vi "ASK_Channelcode.vi"(4 "k":i32, 6 "n":i32, 7 "cod_mode":i32, 8 "error in (no error)":errorcluster caption="错误输入（无错误）", 9 "生产多项式":dbl[](array[numeric]) format="%#_13g", 10 "CRC_Bit":dbl[](array[numeric]) format="%#_13g", 11 "PathIn":path) -> (0 "error out":errorcluster caption="错误输出", 2 "Channel_Bit":dbl[](array[numeric]), 3 "PathOut":path)   [LabVIEW 2015]
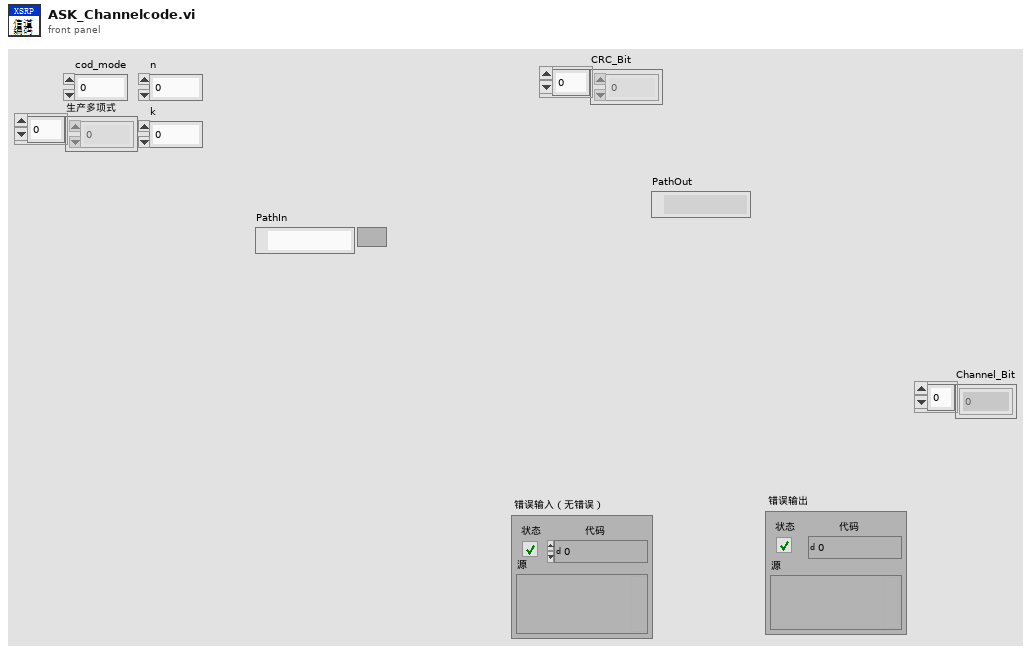
[diagram p1: front panel]
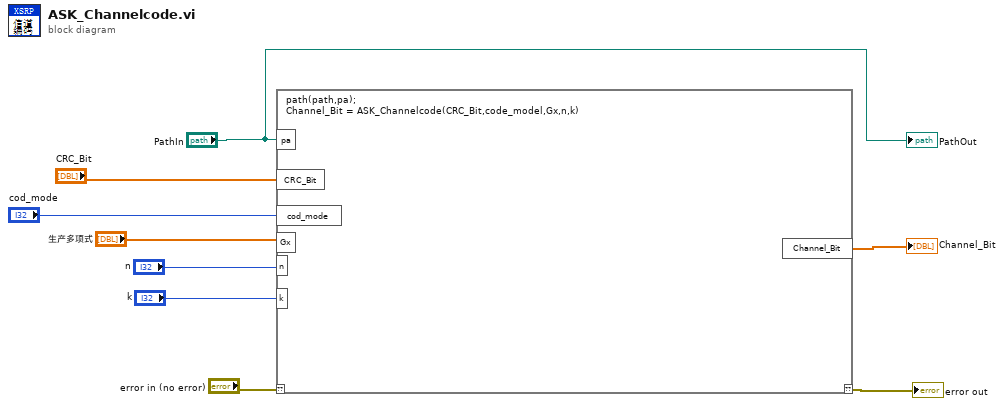
[diagram p0: block diagram]
diagram:
  n1 = script code="path(path,pa);\nChannel_Bit = ASK_Channelcode(CRC_Bit,code_model,Gx,n,k)"("??"="error in (no error)", "pa"="PathIn", "CRC_Bit"="CRC_Bit", "cod_mode"="cod_mode", "Gx"="生产多项式", "n"="n", "k"="k") -> ("??"=→"error out":errorcluster, "Channel_Bit"=→"Channel_Bit":dbl[])
  "PathOut" <- "PathIn"
